vi "DIALOG_Mass Compile.vi"(11 "Quit UE":refnum<user-event>) -> ()   [LabVIEW 2015]
uses:
  Program Files/National Instruments/LabVIEW 2023/user.lib/_OpenG.lib/appcontrol/appcontrol.llb/openg_application_control.lvlib
panel:
  # "Mass compiling BundleMagic"
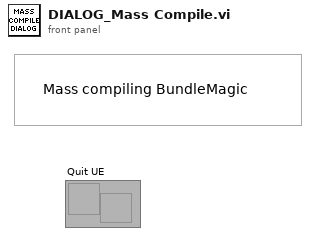
[diagram p1: front panel]
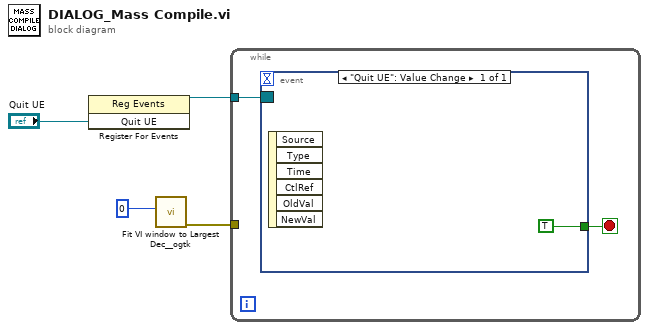
[diagram p0: block diagram]
diagram:
  n1 = register-events("Quit UE") -> (reference out=w3:refnum<event-registration>)  [unwired: 2 in, 1 out]
  n2 = call "Fit VI window to Largest Dec__ogtk.vi"("border spacing (2 px)"=0) -> ("error out"=w2:errorcluster)  [unwired: 5 in, 1 out]
  n3 = while {
    tunnel: w3 -> [w6]
    tunnel: w2 -> [_]
    stop <- w5 stop-if-true
    n4 = event shown="[0] \"Quit UE\": Value Change" {
      selector: w6 -> [_]
      dyn-events: _ -> [_]
      timeout: _ -> [_]
      tunnel: [TRUE] -> w5
      event "Quit UE": Value Change {
        n5 = event-data() -> ()  [unwired: 1 in, 6 out]
      }
    }
  }
